vi "Arrange SubPanels.vi"(8 "错误输入（无错误）":errorcluster, 9 "上窗格":refnum<vi>, 10 "VI引用句柄":refnum<vi>, 11 "rSubPanes":refnum<vi>[](array[refnum])) -> (0 "错误输出":errorcluster)   [LabVIEW 2018, in "MainInterface.lvlib"]
uses:
  MainInterface.lvlib
  <vilib>/Utility/miscctls.llb/LVPositionTypeDef.ctl
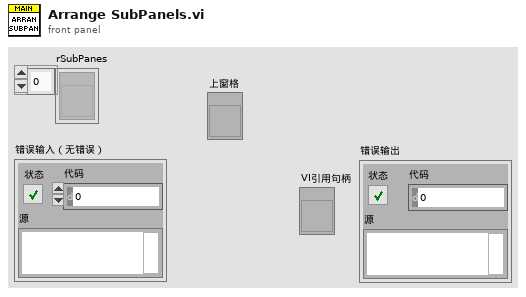
[diagram p1: front panel]
types:
  T1 = typedef "LVPositionTypeDef.ctl" = cluster{"Left":i32, "Top":i32}
  T2 = typedef "LVRectTypeDef.ctl" = cluster{"Left":i16, "Top":i16, "Right":i16, "Bottom":i16}
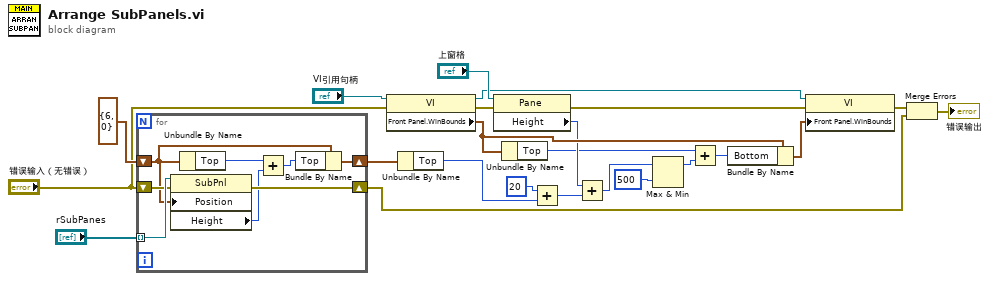
[diagram p0: block diagram]
diagram:
  n1 = for {
    tunnel: "rSubPanes" -> [w31] mode=indexing
    shift-right: [w30] -> w2
    shift-left: T1 {"Left"=6, "Top"=0} ("位置") -> [w26]
    shift-right: [w28] -> w12
    shift-left: "错误输入（无错误）" -> [w29]
    n2 = property class="SubPnl"(reference=w31, error in=w29, "Position"=w26) -> (error out=w28:errorcluster, "Height"=w27:u32)  [unwired: 1 out]
    n3 = Unbundle By Name(w26) -> ("Top"=w25:i32)
    n4 = Add(x=w25, y=w27) -> (x+y=w24:u32)
    n5 = Bundle By Name(cluster=w26, "Top"=w24) -> (w30:T1)
  }
  n6 = property class="VI"(reference="VI引用句柄", error in="错误输入（无错误）") -> (reference out=w19:refnum<vi>, error out=w15:errorcluster, "Front Panel.WinBounds"=w18:T2)
  n7 = Unbundle By Name(w2) -> ("Top"=w1:i32)
  n8 = property class="Pane"(reference="上窗格", error in=w15) -> (error out=w14:errorcluster, "Height"=w8:u32)  [unwired: 1 out]
  n9 = Unbundle By Name(w18) -> ("Top"=w5:i16)
  n10 = Add(x=u32 20, y=w1) -> (x+y=w7:u32)
  n11 = Add(x=w8, y=w7) -> (x+y=w6:u32)
  n12 = Max & Min(x=w6, y=u32 500) -> (max(x,y)=w4:u32)  [unwired: 1 out]
  n13 = Add(x=w5, y=w4) -> (x+y=w3:u32)
  n14 = Bundle By Name(cluster=w18, "Bottom"=w3) -> (w17:T2)
  n15 = property class="VI"(reference=w19, error in=w14, "Front Panel.WinBounds"=w17) -> (error out=w13:errorcluster)  [unwired: 1 out]
  n16 = Merge Errors(w13, w12) -> (→"错误输出":errorcluster)
